vi "PH_PPMA_PowerUnit.Action Seq SM.vi"(0 "VI in":refnum<vi>, 5 "error in (no error)":errorcluster) -> (14 "VI out":refnum<vi>, 19 "error out":errorcluster)   [LabVIEW 2014, in "PH_PPMA_PowerUnit.lvlib"]
uses:
  PH_PPMA_PowerUnit.lvlib
  PH_PowerUnit_BaseClass/PH_PowerUnit_BaseClass.SM States.ctl
  PH_PowerUnit_BaseClass/PH_PowerUnit_BaseClass.lvlib
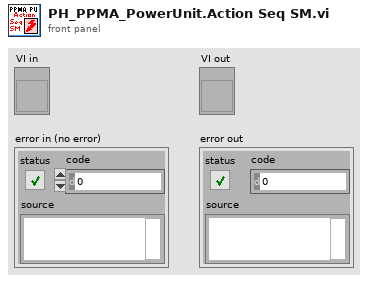
[diagram p1: front panel]
types:
  T1 = typedef "PH_PowerUnit_BaseClass.lvlib/PH_PowerUnit_BaseClass.i attribute.ctl" = cluster{"Constructor finished":bool, "PU":cluster{"In use":bool, "Service ID in use":i32, "GUI Ref":refnum<vi>}, "Enabling":cluster{"State":T2, "GUI Ref":refnum<vi>}, "Timing":cluster{"Last Shot":dbl, "Time between Shots [Sec]":dbl, "Waiting Time over?":bool, "Service ID Waiting Time":i32, "GUI Ref":refnum<vi>, "Instance":cluster{"Status":T3, "linked?":bool, "GUI Ref":refnum<vi>}}, "Sequencer":cluster{"SM State":string, "GUI Ref":refnum<vi>, "linked":bool}, "Subscribed Trendmssgs":cluster{"Tagname":string, "Status":T3, "linked?":bool, "Shot Condition":T3, "GUI Ref":refnum<vi>}[], "PP PU":T4, "Default Voltage (V)":dbl, "GUI Refs":T5, "PSDB data":cluster{"Shot Voltage [V]":dbl, "State TO SM":T6, "Write 2 early":bool}, "State TO SM":T6}
  T2 = typedef "PH_SystemInformation.lvlib/PH_SystemInformationEnabling State.ctl" = i32
  T3 = typedef "PH_StatusHandler.lvlib/PH_StatusHandler.Status.ctl" = i16
  T4 = typedef "PH_PP_Common.lvlib/PH_PP_Common.PUs.ctl" = enum16{"no Info", "PA-19mm-1", "PA-19mm-2", "PA-45mm-PILC", "PA-45mm-MAIN", "MA-PU-1", "MA-PU-2", "MA-PU-3", "MA-PU-4", "MA-PU-5", "MA-PU-6", "MA-FR", "MA-PILC", "PA-45mm-DP"}
  T5 = typedef "PH_PowerUnit_BaseClass.lvlib/PH_PowerUnit_BaseClass.GUI Refs.ctl" = cluster{"Delete Inst":refnum<vi>, "State TO SM":refnum<vi>, "State SM":refnum<vi>, "Fire":refnum<vi>}
  T6 = typedef "PH_PowerUnit_BaseClass.lvlib/PH_PowerUnit_BaseClass.SM States.ctl" = enum16{".", "Stand by", "Switch PU on", "Configure", "Set Default Voltage", "Set STANDBY", "Set READY", "Wait for Shot Cmd", "Open Dump Rods", "Open Ross Relais", "Close Ross Relais", "Switch PSU on", "Switch PSU off", "Charge", "Switch GD Channel on", "Close Dump Rods", "Rods-TO", "RR-TO", "PSU-TO", "Trigger-TO"}
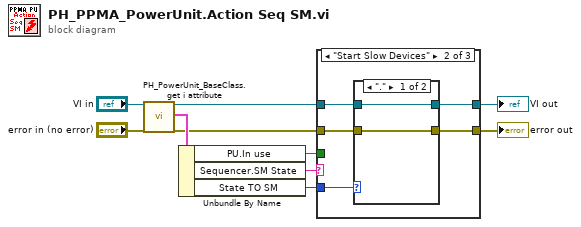
[diagram p0: block diagram]
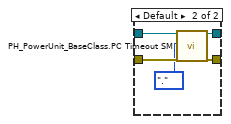
[diagram p3: hidden frame]
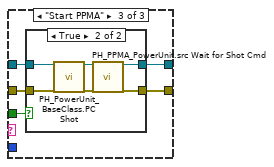
[diagram p4: hidden frame]
diagram:
  n1 = call "PH_PowerUnit_BaseClass.get i attribute.vi"("i ref in"="VI in", "error in (no error)"="error in (no error)") -> ("i ref out"=w3:refnum<vi>, "i attribute"=w8:T1, "error out"=w2:errorcluster)  [unwired: 15 in]
  n2 = Unbundle By Name(w8) -> ("PU.In use"=w4:bool, "Sequencer.SM State"=w5:string, "State TO SM"=w1:T6)
  n3 = case shown="\"Start Slow Devices\"" w5 {
    tunnel: w3 -> [w12 w14 w29]
    tunnel: w2 -> [w11 w13 w27]
    tunnel: [w11 w17 w26] -> w7
    tunnel: [w12 w16 w28] -> w6
    tunnel: w4 -> [_ _ w25]
    tunnel: w1 -> [_ w15 _]
    frame Default {
    }
    frame "Start Slow Devices" {
      n4 = case shown="\".\"" w15 {
        tunnel: [w18 w24] -> w17
        tunnel: [w19 w23] -> w16
        tunnel: w13 -> [w18 w22]
        tunnel: w14 -> [w19 w21]
        frame "." {
        }
        frame Default {
          n5 = call "PH_PowerUnit_BaseClass.PC Timeout SM.vi"("VI in"=w21, "Timeout SM"=PH_PowerUnit_BaseClass.SM_States.".", "error in (no error)"=w22) -> ("VI out"=w23:refnum<vi>, "error out"=w24:errorcluster)  [unwired: 15 in]
        }
      }
    }
    frame "Start PPMA" {
      n6 = case shown="True" w25 {
        tunnel: w29 -> [w31 w37]
        tunnel: [w31 w35] -> w28
        tunnel: w27 -> [w30 w34]
        tunnel: [w30 w32] -> w26
        frame False {
        }
        frame True {
          n7 = call "PH_PowerUnit_BaseClass.PC Shot.vi"("i ref in"=w37, "error in (no error)"=w34) -> ("i ref out"=w36:refnum<vi>, "error out"=w33:errorcluster)  [unwired: 16 in]
          n8 = call "PH_PPMA_PowerUnit.src Wait for Shot Cmd.vi"("i ref in"=w36, "error in (no error)"=w33) -> ("i ref out"=w35:refnum<vi>, "error out"=w32:errorcluster)  [unwired: 16 in]
        }
      }
    }
  }
  "VI out" <- w6
  "error out" <- w7
